vi "Esercitazione 1 - Sottrazioni sequenziali.vi"() -> ()   [LabVIEW 2018]
panel:
  out "Numeric Indicator":i32
  in  "Dial":i32(knob) scale=0.0..10.0
  in  "Knob":i32(knob) scale=0.0..10.0
  in  "Horizontal Fill Slide":i32(slide) scale=0.0..10.0
  in  "Numeric Control":i32
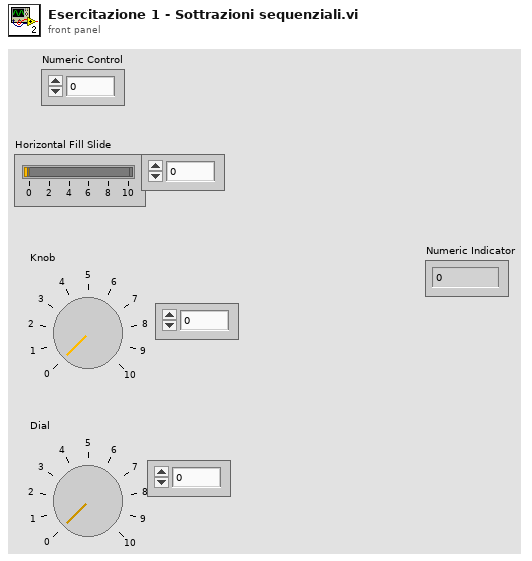
[diagram p1: front panel]
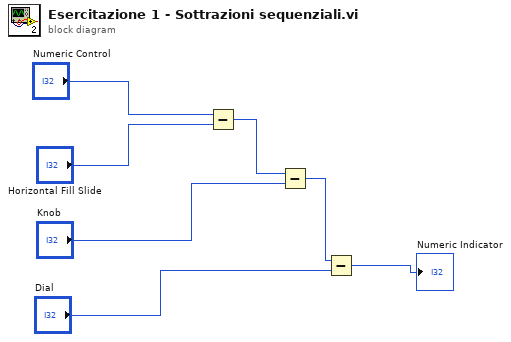
[diagram p0: block diagram]
diagram:
  n1 = Subtract(x="Numeric Control", y="Horizontal Fill Slide") -> (x-y=w4:i32)
  n2 = Subtract(x=w4, y="Knob") -> (x-y=w3:i32)
  n3 = Subtract(x=w3, y="Dial") -> (x-y=→"Numeric Indicator":i32)
